vi "Test Methods.vi"(8 "error in (no error)":errorcluster, 11 "Worker in":refnum<class "Worker.lvclass">) -> (0 "error out":errorcluster, 3 "Worker out":refnum<class "Worker.lvclass">)   [LabVIEW 2024, in "Worker.lvlib" / "Worker.lvclass"]
uses:
  Worker.lvclass
  <vilib>/ActorFramework/Actor/Actor.lvclass/Actor.ctl
  Chef State Logic/Work Logic Messages/Update Count Msg/Update Count Msg.lvclass/Update Count Msg.ctl
  <vilib>/ActorFramework/Message Enqueuer/Message Enqueuer.lvclass/Message Enqueuer.ctl
  <vilib>/ActorFramework/Message Enqueuer/Enqueue.vi
  Chef State Logic/Work Logic Messages/Update Count Msg/Update Count Msg.lvclass
  <vilib>/ActorFramework/Message Priority Queue/Priority Enqueue.vi
  Worker.lvclass/Worker.ctl
  <vilib>/ActorFramework/Actor/Actor.lvclass
  Chef State/Work Messages/Update Count Msg/Update Count Msg.lvclass
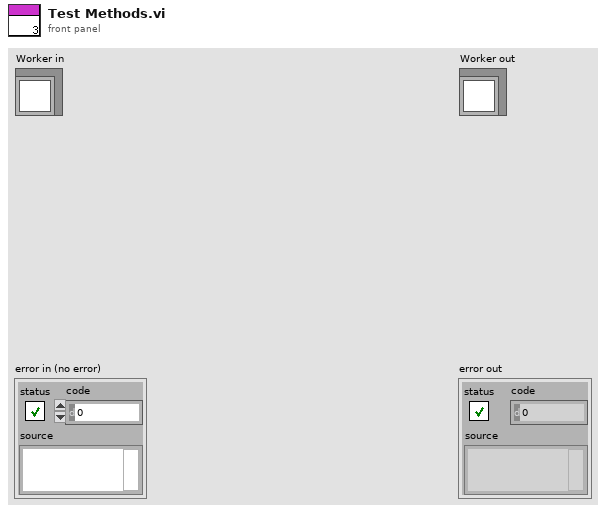
[diagram p1: front panel]
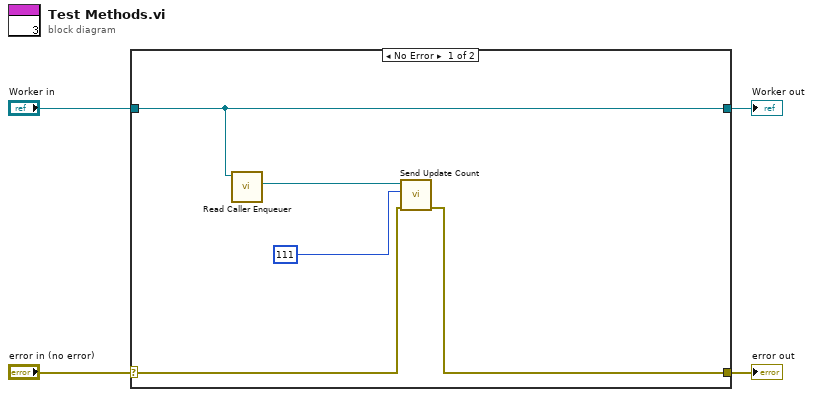
[diagram p0: block diagram]
diagram:
  n1 = case shown="No Error" "error in (no error)" {
    selector: "error in (no error)" -> [w6 w11]
    tunnel: [w5 w11] -> w3
    tunnel: [w9 w10] -> w1
    tunnel: "Worker in" -> [w9 w10]
    frame No Error {
      n2 = call <vilib>:"Read Caller Enqueuer.vi"("Actor"=w9) -> ("Caller Enqueuer"=w8:refnum<class "Message Enqueuer.lvclass">)  [unwired: 10 in]
      n3 = call "Send Update Count.vi"("error in (no error)"=w6, "Count"=u64 111, "Message Enqueuer"=w8) -> ("error out"=w5:errorcluster)  [unwired: 7 in, 1 out]
    }
    frame Error {
    }
  }
  "error out" <- w3
  "Worker out" <- w1
